vi "Yi.vi"(8 "error in (no error)":errorcluster, 11 "cam 0":T1) -> (0 "error out":errorcluster, 3 "output cluster":T1={"incident ANGLE COMPENSATION"=[], "dp/B [MeV/C/B]"=[], "charge compensation"=[], "Momentum [MeV/C]"=[], "energyDependence Input"=[], "pixel angle (y)"=[], "dp [MeV/C/] "=[], "angle 2Dfor spectrumj"=[], "dp [MeV/C] 2D"=[], "charge compensation 2D"=[], "Screen&Camera 2"={"Screen Orientation"="Regular", "Screen angle"="Flat", "Lens"=enum."FL1-f8x08", "Calibration (mm/pix)"=1.0}, "ROI info"={"npix-X"=0, "npix-Y"=0, "Left [pix]"=0.0, "Top [pix]"=0.0}, "Y 2D full angle"=[], "calib pixel"={"y1(pixel)"=[], "y2(pixel)"=[], "dp/B [MeV/C/B] (pixel)"=[], "energyDependence Input(pixel)"=[], "bending angle [deg](pixel)"=[], "total path(pixel)"=[], "pixel angle (y)(pixel)"=[], "energy dependence (pixel)"=[], "charge compensation (pixel)"=[], "Momentum [MeV/C](pixel)"=[], "angular compensation(pixel)"=[]}, "2D"={"dp"=[], "chargeCompensation"=[], "angle"=[], "Momentum"=[]}, "UserROI"={"Width"=0.0, "Hight"=0.0, "OffsetX"=0.0, "OffsetY"=0.0}, "final"={"X"=[], "xi"=[], "delta momentum"=0.0, "Y"=[], "yi"=[], "angle (Y)"=[], "delta angle"=0.0, "scale delta angle"=0.0, "intraX"=0.0, "intraY"=0.0, "mask"=[]}, "B[T]"=0.0, "index"=0.0})   [LabVIEW 2013]
uses:
  calib_Sub_Typdef.ctl
  ScreenCam2_TypDEf.ctl
  CamAndObj_TypDEf.ctl
  ROIInfo_TypDef.ctl
  calibPixel.ctl
  2DTypDef.ctl
  CamRoiTypDef.ctl
  finalCalibTypdef.ctl
  <vilib>/gmath/NI_Gmath.lvlib
panel:
  out "max value":dbl
  out "Waveform Graph":dbl[](graph)
  out "ceil(x): smallest int >= x":dbl
  out "final.Y":dbl[][](graph)
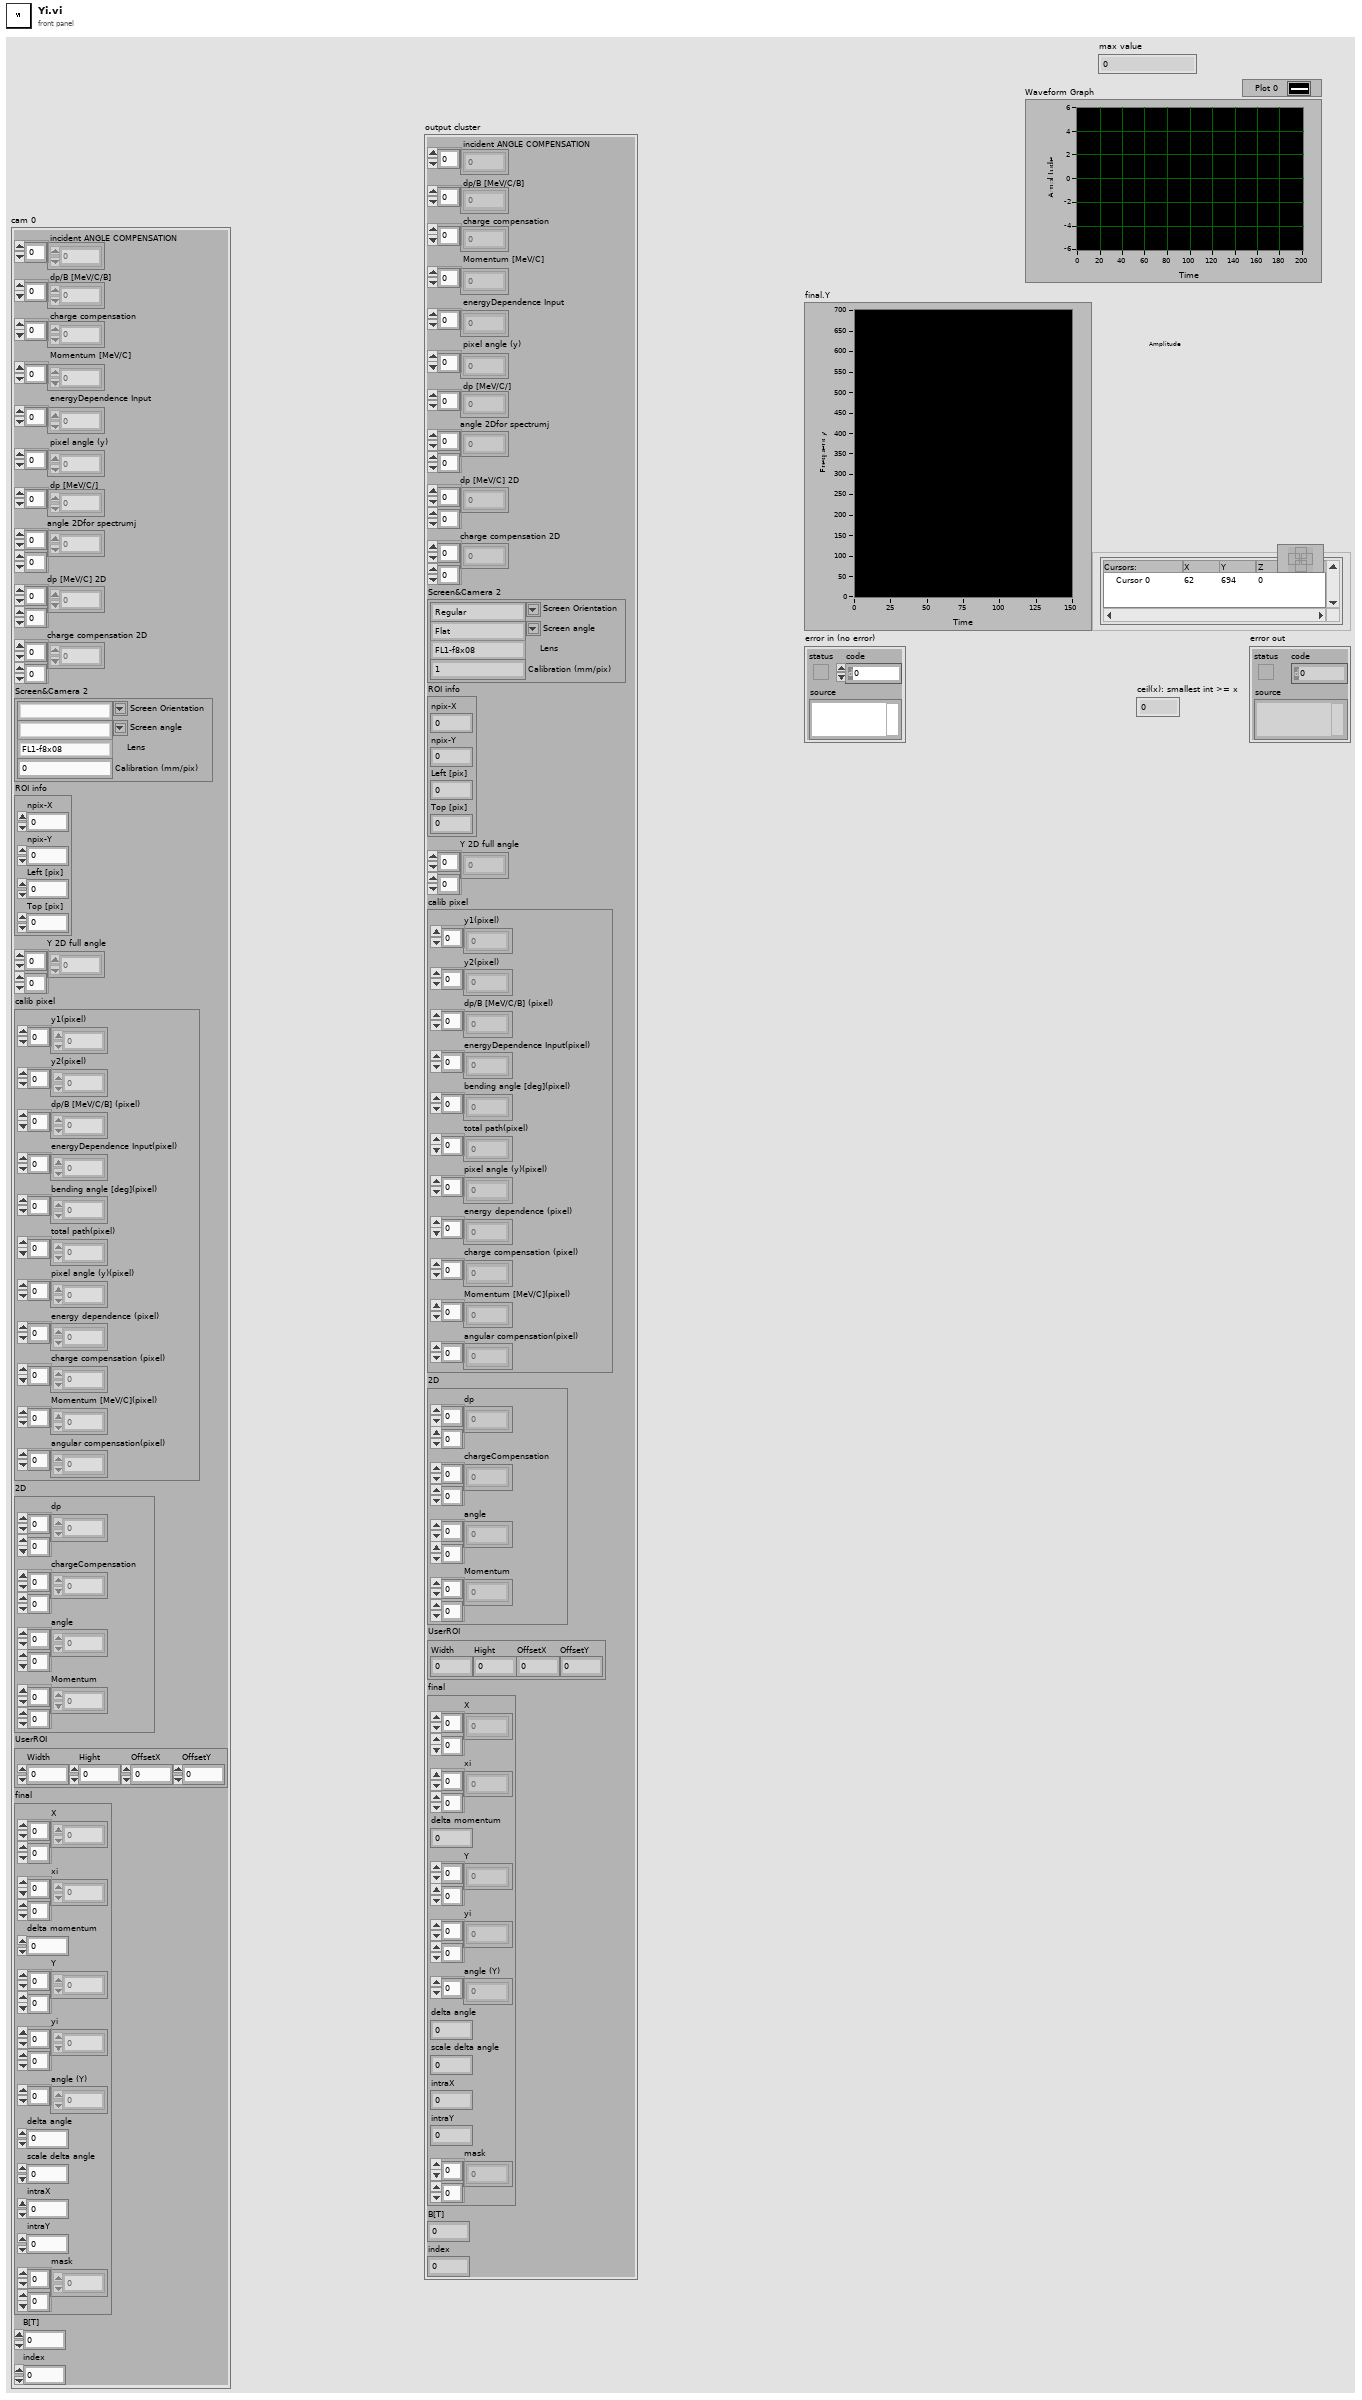
[diagram p1: front panel]
types:
  T1 = typedef "calib_Sub_Typdef.ctl" = cluster{"incident ANGLE COMPENSATION":dbl[], "dp/B [MeV/C/B]":dbl[], "charge compensation":dbl[], "Momentum [MeV/C]":dbl[], "energyDependence Input":dbl[], "pixel angle (y)":dbl[], "dp [MeV/C/] ":dbl[], "angle 2Dfor spectrumj":dbl[][], "dp [MeV/C] 2D":dbl[][], "charge compensation 2D":dbl[][], "Screen&Camera 2":T2, "ROI info":T4, "Y 2D full angle":dbl[][], "calib pixel":T5, "2D":T6, "UserROI":T7, "final":T8, "B[T]":dbl, "index":dbl}
  T2 = typedef "ScreenCam2_TypDEf.ctl" = cluster{"Screen Orientation":string, "Screen angle":string, "Lens":T3, "Calibration (mm/pix)":dbl}
  T3 = typedef "CamAndObj_TypDEf.ctl" = enum16{"FL1-f8x08", "FL1-f8x06", "FL1-f8", "ch300-f50", "FL2G-f8", "FL3M14-f8", "FL3M14-f8x08", "FL3M14-f8x08(2x2)"}
  T4 = typedef "ROIInfo_TypDef.ctl" = cluster{"npix-X":i32, "npix-Y":i32, "Left [pix]":dbl, "Top [pix]":dbl}
  T5 = typedef "calibPixel.ctl" = cluster{"y1(pixel)":dbl[], "y2(pixel)":dbl[], "dp/B [MeV/C/B] (pixel)":dbl[], "energyDependence Input(pixel)":dbl[], "bending angle [deg](pixel)":dbl[], "total path(pixel)":dbl[], "pixel angle (y)(pixel)":dbl[], "energy dependence (pixel)":dbl[], "charge compensation (pixel)":dbl[], "Momentum [MeV/C](pixel)":dbl[], "angular compensation(pixel)":dbl[]}
  T6 = typedef "2DTypDef.ctl" = cluster{"dp":dbl[][], "chargeCompensation":dbl[][], "angle":dbl[][], "Momentum":dbl[][]}
  T7 = typedef "CamRoiTypDef.ctl" = cluster{"Width":dbl, "Hight":dbl, "OffsetX":dbl, "OffsetY":dbl}
  T8 = typedef "finalCalibTypdef.ctl" = cluster{"X":dbl[][], "xi":dbl[][], "delta momentum":dbl, "Y":dbl[][], "yi":dbl[][], "angle (Y)":dbl[], "delta angle":dbl, "scale delta angle":dbl, "intraX":dbl, "intraY":dbl, "mask":dbl[][]}
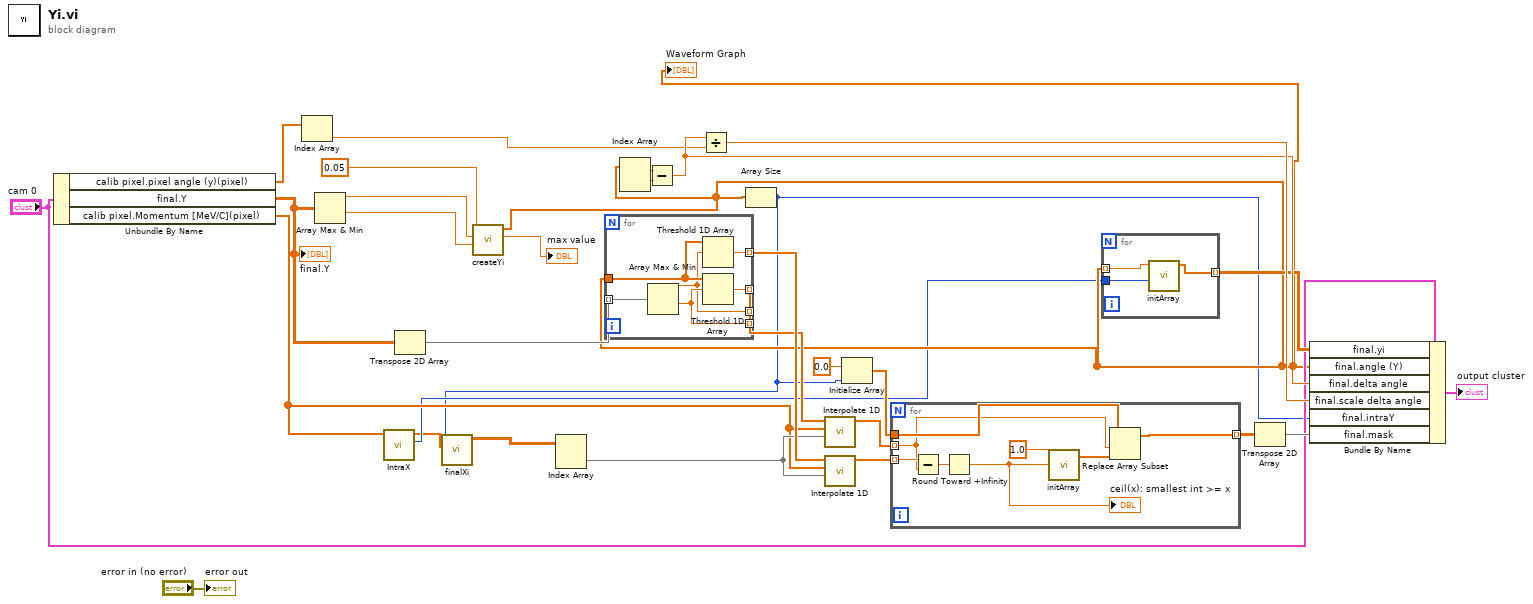
[diagram p0: block diagram]
diagram:
  n1 = Unbundle By Name("cam 0") -> ("calib pixel.pixel angle (y)(pixel)"=w31:dbl[], "final.Y"=w12:dbl[][], "calib pixel.Momentum [MeV/C](pixel)"=w7:dbl[])
  "final.Y" <- w12
  n2 = Index Array(array=w31) -> (element=w26:dbl)  [unwired: 1 in]
  n3 = Array Max & Min(array=w12) -> (max value=w25:dbl, min value=w9:dbl)  [unwired: 2 out]
  n4 = call "IntraX.vi"("Momentum [MeV/C](pixel)"=w7) -> ("IntraX"=w6:i32, "Ramp Pattern"=w5:dbl[])  [unwired: 7 in, 2 out]
  n5 = Transpose 2D Array(2D array=w12) -> (transposed array=w22:dbl[][])
  n6 = call "createYi.vi"("Min"=w9, "Max"=w25, "delta"=0.05) -> ("max value"=→"max value":dbl, "Array"=w10:dbl[])  [unwired: 7 in]
  "Waveform Graph" <- w10
  n7 = for {
    tunnel: w22 -> [w37] mode=indexing
    tunnel: [w35] -> w21 mode=indexing
    tunnel: [w34] -> w20 mode=indexing
    tunnel: w10 -> [w36]
    tunnel: [w33] -> _ mode=indexing
    tunnel: [w32] -> _ mode=indexing
    n8 = Array Max & Min(array=w37) -> (max value=w32:dbl, min value=w33:dbl)  [unwired: 2 out]
    n9 = Threshold 1D Array(2:w32, 3:w36) -> (0:w35:dbl)  [unwired: 1 in]
    n10 = Threshold 1D Array(2:w33, 3:w36) -> (0:w34:dbl)  [unwired: 1 in]
  }
  n11 = Index Array(array=w10) -> (element #1=w27:dbl, element #2=w28:dbl)  [unwired: 2 in]
  n12 = Subtract(x=w28, y=w27) -> (x-y=w29:dbl)
  n13 = Divide(x=w29, y=w26) -> (x/y=w30:dbl)
  n14 = Array Size(array=w10) -> (size(s)=w4:i32)
  n15 = call "finalXi.vi"("Ramp Pattern"=w5, "intraY"=w4) -> ("Array"=w3:dbl[][])  [unwired: 9 in]
  n16 = Index Array(array=w3) -> (element=w13:dbl[])  [unwired: 2 in]
  n17 = call <vilib>:"Interpolate 1D.vi"("xi"=w13, "X"=w7, "Y"=w20) -> ("yi"=w17:dbl[])  [unwired: 6 in, 2 out]
  n18 = call <vilib>:"Interpolate 1D.vi"("xi"=w13, "X"=w7, "Y"=w21) -> ("yi"=w16:dbl[])  [unwired: 6 in, 2 out]
  n19 = Initialize Array(0.0 ("element"), w4) -> (w18:dbl[])
  n20 = for {
    tunnel: w17 -> [w41] mode=indexing
    tunnel: w18 -> [w42]
    tunnel: w16 -> [w45] mode=indexing
    tunnel: [w39] -> w15 mode=indexing
    n21 = Subtract(x=w45, y=w41) -> (x-y=w44:dbl)
    n22 = Round Toward +Infinity(x=w44) -> (ceil(x): smallest int >= x=w38:dbl)
    "ceil(x): smallest int >= x" <- w38
    n23 = call "initArray.vi"("dim"=w38, "element"=1.0) -> ("Array"=w40:dbl[])  [unwired: 9 in]
    n24 = Replace Array Subset(array=w42, new element=w40, index=w41) -> (w39:dbl[])
  }
  n25 = for {
    tunnel: w10 -> [w48] mode=indexing
    tunnel: w6 -> [w47]
    tunnel: [w46] -> w23 mode=indexing
    n26 = call "initArray.vi"("dim"=w47, "element"=w48) -> ("Array"=w46:dbl[])  [unwired: 9 in]
  }
  n27 = Transpose 2D Array(2D array=w15) -> (transposed array=w14:dbl[][])
  n28 = Bundle By Name(cluster="cam 0", "final.yi"=w23, "final.angle (Y)"=w10, "final.delta angle"=w29, "final.scale delta angle"=w30, "final.intraY"=w4, "final.mask"=w14) -> (→"output cluster":T1)
  "error out" <- "error in (no error)"
